vi "ma_put 2.vi"(8 "Error":errorcluster, 10 "初始進入":bool[][](array[boolean]), 11 "KNR in":T1) -> (0 "error out 4":errorcluster caption="error out", 2 "最終堆疊版 2":bool[][](array[boolean]), 3 "KNR out":T1, 5 "x2":dbl)   [LabVIEW 2013]
uses:
  <userlib>/KNR OS 3.0 LabVIEW Toolkit/Type Definition/KNR3 Reference.ctl
  <userlib>/_FPGA Interface Advanced Tools/FPGA Interface Base/FPGA Interface Base.lvclass
  <userlib>/KNR OS 3.0 LabVIEW Toolkit/Type Definition/Resource.ctl
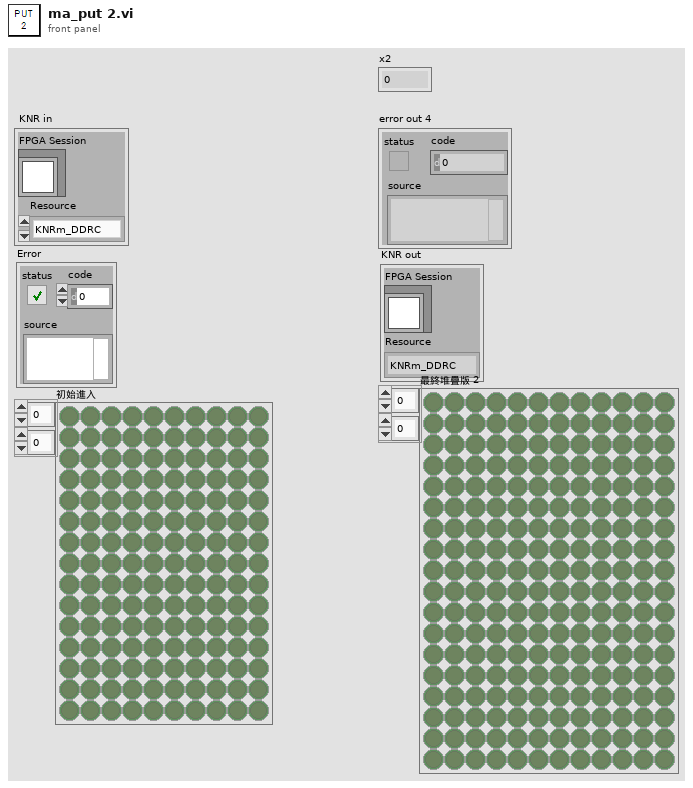
[diagram p1: front panel]
types:
  T1 = typedef "KNR3 Reference.ctl" = cluster{"FPGA Session":refnum<class "FPGA Interface Base.lvclass">, "Resource":T2}
  T2 = typedef "Resource.ctl" = enum16{"KNRm_DDRC", "KNRm_DDDD", "KNRm_DDDR", "KNRm_DDDC", "KNR"}
  T3 = cluster{"Position":cluster{"X":sgl, "Y":sgl}, "Radius":dbl, "Score":dbl}[]
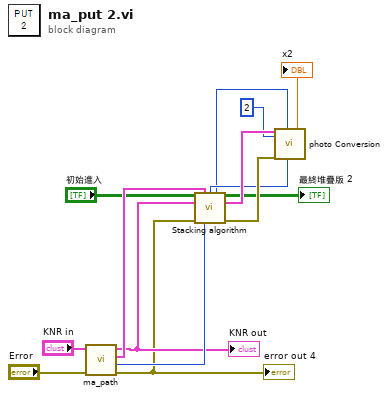
[diagram p0: block diagram]
diagram:
  n1 = call "ma_path.vi"("Error"="Error", "KNR in"="KNR in") -> ("error out 4"=w9:errorcluster, "Number of Matches (Shape Detection 1)"=w11:i32, "Circles (Shape Detection 1)"=w12:T3, "KNR out"=w10:T1)  [unwired: 4 in, 2 out]
  "error out 4" <- w9
  "KNR out" <- w10
  n2 = call "Stacking algorithm.vi"("初始進入"="初始進入", "Circles (Shape Detection 1) 2"=w12, "KNR in"=w10, "Error"=w9, "ふ计"=w11) -> ("底盤T數"=w5:i32, "X"=w4:i32, "最終堆疊版 2"=→"最終堆疊版 2":bool[][], "KNR out"=w8:T1, "error out"=w7:errorcluster)  [unwired: 1 in, 5 out]
  n3 = call "photo Conversion.vi"("KNR in"=w8, "順序"=2, "error in"=w7, "x2"=w4, "t2"=w5) -> ("x"=→"x2":dbl)  [unwired: 12 in, 2 out]
